vi "CSV Reader.vi"(6 "Reset":bool, 7 "Index in":i32, 10 "Parcel Length":i32, 11 "Config":T2={"Mode"=enum."Full timestamp", "delimiter (\\t)"="\t", "Path"=path "", "Rectangular?"=FALSE}) -> (1 "Analog":dbl[][](array[numeric]), 2 "Complex":cdb[][](array[numeric]), 3 "Timestamps":timestamp[](array[timestamp]), 4 "EOF?":bool, 5 "Index out":i32)   [LabVIEW 2017]
uses:
  Mode CSV reader.ctl
  <vilib>/Utility/file.llb/Read Delimited Spreadsheet (DBL).vi
  <vilib>/Utility/file.llb/Read Delimited Spreadsheet (string).vi
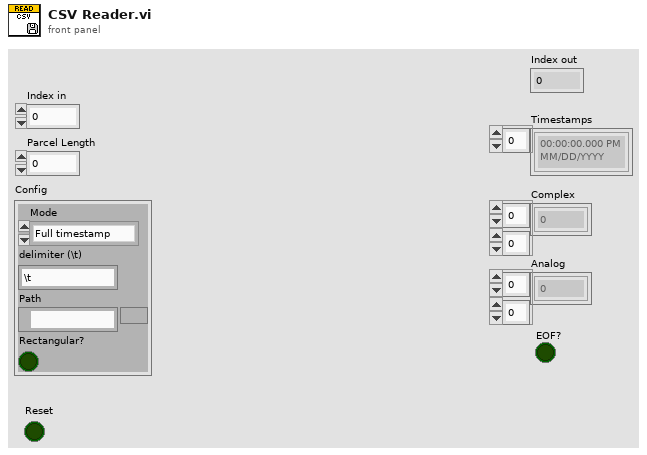
[diagram p1: front panel]
types:
  T1 = typedef "Mode CSV reader.ctl" = enum16{"Full timestamp", "Relative Time", "Seconds Time"}
  T2 = cluster{"Mode":T1, "delimiter (\\t)":string, "Path":path, "Rectangular?":bool}
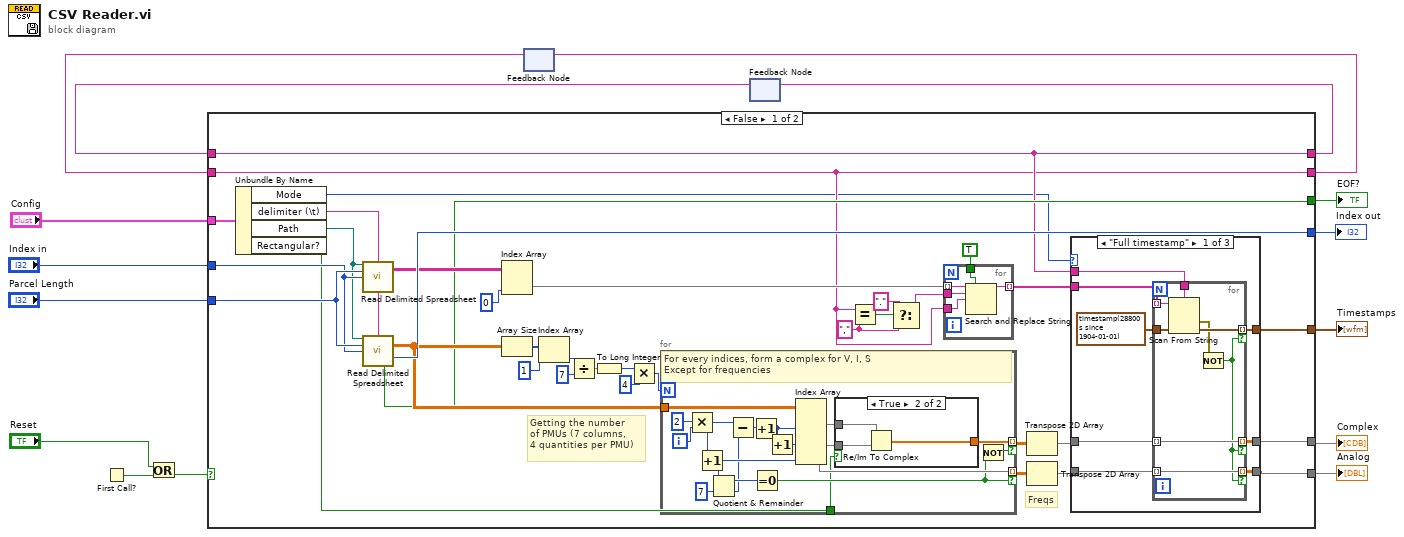
[diagram p0: block diagram]
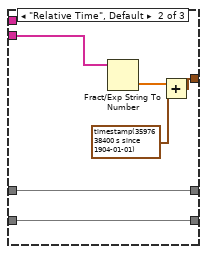
[diagram p2: hidden frame]
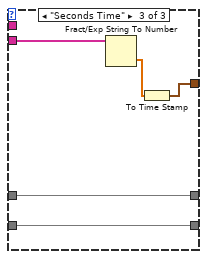
[diagram p3: hidden frame]
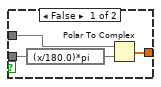
[diagram p4: hidden frame]
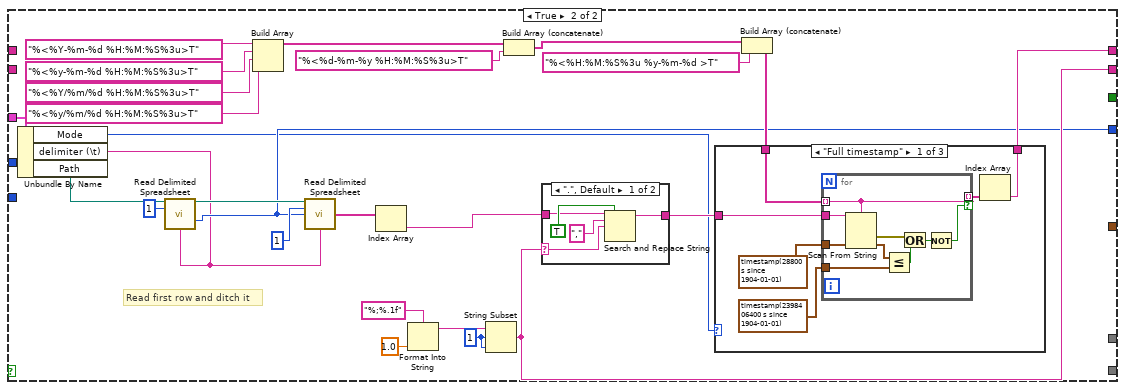
[diagram p5: hidden frame]
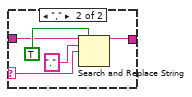
[diagram p8: hidden frame]
diagram:
  n1 = First Call?() -> (First Call?: T/F=w15:bool)
  n2 = Or(x="Reset", y=w15) -> (x .or. y?=w4:bool)
  n3 = feedback #1() -> (w11:string)  [unwired: 1 in]
  n4 = feedback #2() -> (w13:string)  [unwired: 1 in]
  n5 = case shown="False" w4 {
    tunnel: [w35 w126] -> w14
    tunnel: w13 -> [w35 _]
    tunnel: [w27 w116] -> w12
    tunnel: w11 -> [w27 _]
    tunnel: [w49 w113] -> w10
    tunnel: "Index in" -> [w50 _]
    tunnel: "Parcel Length" -> [w51 _]
    tunnel: [w39 _] -> w7
    tunnel: [w36 _] -> w6
    tunnel: "Config" -> [w26 w112]
    tunnel: [w21 _] -> w1
    tunnel: [w20 _] -> w2
    frame False {
      w29 = "," ("search string")
      # "Freqs"
      # "Getting the number\nof PMUs (7 columns, \n4 quantities per PMU)"
      n6 = Unbundle By Name(w26) -> ("Mode"=w25:T1, "delimiter (\\t)"=w24:string, "Path"=w23:path, "Rectangular?"=w22:bool)
      n7 = call-poly <vilib>:"Read Delimited Spreadsheet.vi"("file path (dialog if empty)"=w23, "number of rows (all:-1)"=w51, "start of read offset (chars.:0)"=w50, "delimiter (\\t)"=w24) -> ("all rows"=w38:string[][])  [unwired: 6 in, 5 out]
      n8 = call-poly <vilib>:"Read Delimited Spreadsheet.vi"("file path (dialog if empty)"=w23, "number of rows (all:-1)"=w51, "start of read offset (chars.:0)"=w50, "delimiter (\\t)"=w24) -> ("all rows"=w40:dbl[][], "mark after read (chars.)"=w49:i32, "EOF?"=w36:bool)  [unwired: 6 in, 3 out]
      n9 = Index Array(array=w38, index (col)=0 ("disabled index (col)")) -> (element=w34:string[])  [unwired: 1 in]
      n10 = Array Size(array=w40) -> (size(s)=w43:i32[])
      n11 = Index Array(array=w43, index=1) -> (element=w45:i32)
      n12 = Divide(x=w45, y=7) -> (x/y=w47:dbl)
      n13 = To Long Integer(number=w47) -> (32bit integer=w41:i32)
      n14 = Multiply(x=w41, y=4) -> (x*y=w42:i32)
      n15 = for {
        N: w42 -> [_]
        tunnel: [w99] -> w19 mode=indexing if=w89
        tunnel: w40 -> [w96]
        tunnel: [w90] -> w18 mode=indexing if=w88
        tunnel: w22 -> [w84]
        i -> [w92]
        # "For every indices, form a complex for V, I, S\nExcept for frequencies"
        n16 = Multiply(x=2, y=w92) -> (x*y=w85:i32)
        n17 = Increment(x=w85) -> (x+1=w91:i32)
        n18 = Quotient & Remainder(x=w91, y=7) -> (x-y*floor(x/y)=w93:i32, floor(x/y)=w86:i32)
        n19 = Subtract(x=w85, y=w86) -> (x-y=w87:i32)
        n20 = Increment(x=w87) -> (x+1=w97:i32)
        n21 = Equal To 0?(x=w93) -> (x = 0?=w88:bool)
        n22 = Increment(x=w97) -> (x+1=w95:i32)
        n23 = Index Array(array=w96, index (col) #1=w97, index (col) #2=w95, index (col) #3=w91) -> (element #1=w100:dbl[], element #2=w101:dbl[], element #3=w90:dbl[])  [unwired: 3 in]
        n24 = case shown="True" w84 {
          tunnel: w101 -> [w104 w108]
          tunnel: w100 -> [w103 w107]
          tunnel: [w105 w106] -> w99
          frame False {
            n25 = expression code="(x/180.0)*pi" ("degrees to radians")(w104) -> (w102:dbl[])
            n26 = Polar To Complex(1:w102, 2:w103) -> (0:w105:cdb[])
          }
          frame True {
            n27 = Re/Im To Complex(1:w108, 2:w107) -> (0:w106:cdb[])
          }
        }
        n28 = Not(x=w88) -> (.not. x?=w89:bool)
      }
      n29 = Equal?(x=w27, y=w29) -> (x = y?=w28:bool)
      n30 = Select(t="." ("search string"), s=w28, f=w29) -> (s? t:f=w30:string)
      n31 = for {
        tunnel: w34 -> [w56] mode=indexing
        tunnel: [w55] -> w33 mode=indexing
        tunnel: w27 -> [w53]
        tunnel: TRUE ("replace all? (F)") -> [w54]
        tunnel: w30 -> [w52]
        n32 = Search and Replace String(replace all?=w54, input string=w56, search string=w52, replace string=w53) -> (result string=w55:string)  [unwired: 4 in, 3 out]
      }
      n33 = Transpose 2D Array(2D array=w19) -> (transposed array=w17:cdb[][])
      n34 = Transpose 2D Array(2D array=w18) -> (transposed array=w16:dbl[][])
      n35 = case shown="\"Full timestamp\"" w25 {
        tunnel: [w63 w77 w81] -> w39
        tunnel: w33 -> [w62 w76 w83]
        tunnel: w35 -> [w61 _ _]
        tunnel: w17 -> [w60 w74 w80]
        tunnel: w16 -> [w59 w73 w79]
        tunnel: [w58 w74 w80] -> w21
        tunnel: [w57 w73 w79] -> w20
        frame "Full timestamp" {
          n36 = for {
            tunnel: w61 -> [w72]
            tunnel: timestamp(28800 s since 1904-01-01) ("default value 1") -> [w71]
            tunnel: [w70] -> w63 mode=indexing if=w65
            tunnel: w62 -> [w69] mode=indexing
            tunnel: w60 -> [w68] mode=indexing
            tunnel: w59 -> [w67] mode=indexing
            tunnel: [w68] -> w58 mode=indexing if=w65
            tunnel: [w67] -> w57 mode=indexing if=w65
            n37 = Scan From String(format string=w72, input string=w69, default 1=w71) -> (error out=w66:errorcluster, output 1=w70:timestamp)  [unwired: 2 in, 2 out]
            n38 = Not(x=w66) -> (.not. x?=w65:bool)
          }
        }
        frame "Relative Time", Default {
          n39 = Fract/Exp String To Number(string=w76) -> (number=w75:dbl[])  [unwired: 3 in, 1 out]
          n40 = Add(x=w75, y=timestamp(3597638400 s since 1904-01-01) ("default value 1")) -> (x+y=w77:timestamp[])
        }
        frame "Seconds Time" {
          n41 = Fract/Exp String To Number(string=w83) -> (number=w82:dbl[])  [unwired: 3 in, 1 out]
          n42 = To Time Stamp(1:w82) -> (0:w81:timestamp[])
        }
      }
    }
    frame True {
      w117 = 1 ("offset (0)")
      # "Read first row and ditch it"
      n43 = Unbundle By Name(w112) -> ("Mode"=w111:T1, "delimiter (\\t)"=w109:string, "Path"=w110:path)
      n44 = call-poly <vilib>:"Read Delimited Spreadsheet.vi"("file path (dialog if empty)"=w110, "number of rows (all:-1)"=1, "delimiter (\\t)"=w109) -> ("new file path (Not A Path if cancelled)"=w128:path, "mark after read (chars.)"=w113:i32)  [unwired: 7 in, 4 out]
      n45 = Build Array("%<%Y-%m-%d %H:%M:%S%3u>T", "%<%y-%m-%d %H:%M:%S%3u>T", "%<%Y/%m/%d %H:%M:%S%3u>T", "%<%y/%m/%d %H:%M:%S%3u>T") -> (w125:string[])
      n46 = call-poly <vilib>:"Read Delimited Spreadsheet.vi"("file path (dialog if empty)"=w128, "number of rows (all:-1)"=1, "start of read offset (chars.:0)"=w113, "delimiter (\\t)"=w109) -> ("first row"=w127:string[])  [unwired: 6 in, 5 out]
      n47 = Index Array(array=w127) -> (element=w114:string)  [unwired: 1 in]
      n48 = Format Into String(format string="%;%.1f", 1.0 ("input 1")) -> (resulting string=w118:string)  [unwired: 2 in, 1 out]
      n49 = String Subset(string=w118, offset (0)=w117, length (rest)=w117) -> (substring=w116:string)
      n50 = Build Array (concatenate)(w125, "%<%d-%m-%y %H:%M:%S%3u>T") -> (w123:string[])
      n51 = case shown="\".\", Default" w116 {
        selector: w116 -> [w152 w156]
        tunnel: [w154 w157] -> w115
        tunnel: w114 -> [w150 w155]
        frame ".", Default {
          n52 = Search and Replace String(replace all?=TRUE ("replace all? (F)"), input string=w150, search string=",", replace string=w152) -> (result string=w154:string)  [unwired: 4 in, 3 out]
        }
        frame "," {
          n53 = Search and Replace String(replace all?=TRUE ("replace all? (F)"), input string=w155, search string=".", replace string=w156) -> (result string=w157:string)  [unwired: 4 in, 3 out]
        }
      }
      n54 = Build Array (concatenate)(w123, "%<%H:%M:%S%3u %y-%m-%d >T") -> (w121:string[])
      n55 = case shown="\"Full timestamp\"" w111 {
        tunnel: [w139 _ _] -> w126
        tunnel: w121 -> [w138 _ _]
        tunnel: w115 -> [w137 _ _]
        frame "Full timestamp" {
          n56 = for {
            tunnel: w138 -> [w145] mode=indexing
            tunnel: timestamp(2398406400 s since 1904-01-01) ("default value 1") -> [w149]
            tunnel: [w145] -> w136 mode=indexing if=w142
            tunnel: w137 -> [w144]
            tunnel: timestamp(28800 s since 1904-01-01) ("default value 1") -> [w141]
            n57 = Scan From String(format string=w145, input string=w144, default 1=w141) -> (error out=w148:errorcluster, output 1=w143:timestamp)  [unwired: 2 in, 2 out]
            n58 = Less Or Equal?(x=w143, y=w149) -> (x <= y?=w147:bool)
            n59 = Or(x=w148, y=w147) -> (x .or. y?=w146:bool)
            n60 = Not(x=w146) -> (.not. x?=w142:bool)
          }
          n61 = Index Array(array=w136) -> (element=w139:string)  [unwired: 1 in]
        }
        frame "Relative Time", Default {
        }
        frame "Seconds Time" {
        }
      }
    }
  }
  "Index out" <- w10
  "Timestamps" <- w7
  "Complex" <- w1
  "Analog" <- w2
  "EOF?" <- w6
  n62 = feedback-in #1(w12) -> ()
  n63 = feedback-in #2(w14) -> ()
